vi "I2C Close.vi"(7 "I2C Channel (0)":u8, 8 "Error In":errorcluster, 11 "LINX Resource":T1) -> (0 "Error Out":errorcluster, 3 "LINX Resource":T1)   [LabVIEW 2014, in "LMH-LINX.lvlib"]
doc: "Close the specified I2C channel. Not all devices support or require this fuction. Most Wiring (Arduino) comaptible devices do not support this function. \n\nIf the current device does not support this function it will return a 'Function Not Supported' warning which should be handled by the users code."
uses:
  LMH-LINX.lvlib
  Private/Type Defs/LINX Ref.ctl
  Private/Type Defs/Platform.ctl
  Private/Type Defs/Interface.ctl
  Private/Device/Type Defs/LINX Device Config.ctl
  Private/Device/Type Defs/TCP Config.ctl
  Private/Device/Type Defs/Channels.ctl
  Private/Type Defs/Peripheral.ctl
  Private/Type Defs/Channel FGV States.ctl
  <vilib>/myRIO/Instrument Drivers/Onboard IO/I2C/typedefs/I2C Transfer Rate.ctl
  <vilib>/myRIO/Instrument Drivers/Onboard IO/I2C/I2C.lvlib
  <vilib>/myRIO/Instrument Drivers/Onboard IO/I2C/typedefs/I2C Configuration.ctl
  <vilib>/myRIO/Common/Instrument Driver Framework/myRIO v1.0/I2C/typedefs/I2C Channels Enum.ctl
  <vilib>/myRIO/Common/Instrument Driver Framework/Utilities/typedefs/Generic FPGA Reference.ctl
  <vilib>/myRIO/Common/Instrument Driver Framework/Utilities/typedefs/myRIO v1.0 Reference.ctl
  <vilib>/myRIO/Common/Instrument Driver Framework/Utilities/typedefs/Hardware Version Enum.ctl
  <vilib>/myRIO/Common/Instrument Driver Framework/Utilities/typedefs/myRIO Generic Hardware Reference.ctl
  <vilib>/myRIO/Instrument Drivers/Onboard IO/I2C/typedefs/I2C Reference.ctl
  Private/Device/Device.lvlib
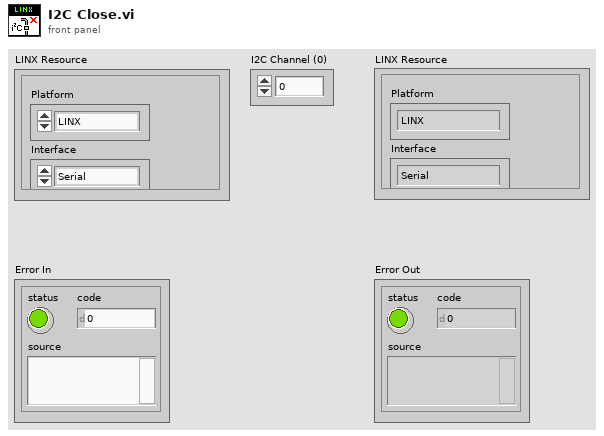
[diagram p1: front panel]
types:
  T1 = typedef "LMH-LINX.lvlib/LINX Ref.ctl" = cluster{"Platform":T2, "Interface":T3, "LINX Device Config":T4}
  T2 = typedef "LMH-LINX.lvlib/Platform.ctl" = enum16{"LINX", "myRIO"}
  T3 = typedef "LMH-LINX.lvlib/Interface.ctl" = enum16{"Serial", "TCP"}
  T4 = typedef "LMH-LINX.lvlib/Device.lvlib/LINX Device Config.ctl" = cluster{"Interface":T3, "COM Port":refnum<visa-resource-name>, "TCP Configuration":T5, "Device Family":u8, "Device ID":u8, "Device Name":string, "TCP Ref":refnum<k5>, "Channels":T6}
  T5 = typedef "LMH-LINX.lvlib/Device.lvlib/TCP Config.ctl" = cluster{"IP Address":string, "Port":u16}
  T6 = typedef "LMH-LINX.lvlib/Channels.ctl" = cluster{"DI":u8[], "DO":u8[], "AI":u8[], "AO":u8[], "PWM":u8[], "QE":u8[], "UART":u8[], "I2C 2":u8[], "SPI":u8[], "CAN":u8[], "Servo":u8[], "AI Ref (V)":dbl, "AO Ref (V)":dbl, "AO Resolution (Bits)":u8}
  T7 = typedef "LMH-LINX.lvlib/Peripheral.ctl" = enum8{"DI", "DO", "AI", "AO", "PWM", "QE", "UART", "I2C", "SPI", "CAN", "Servo"}
  T8 = typedef "LMH-LINX.lvlib/Channel FGV States.ctl" = enum16{"Initialize", "Get", "Set"}
  T9 = typedef "I2C.lvlib/I2C Reference.ctl" = cluster{"myRIO Reference":T10, "I2C Channels Enum":T14, "I2C Configuration":T15}
  T10 = typedef "myRIO Generic Hardware Reference.ctl" = cluster{"myRIO Model":T11, "myRIO Hardware Reference":T12}
  T11 = typedef "Hardware Version Enum.ctl" = enum16{"Unknown", "myRIO-1900", "myRIO-1950"}
  T12 = typedef "myRIO v1.0 Reference.ctl" = cluster{"Generic FPGA Reference":T13, "Allow multiple opens":bool}
  T13 = typedef "Generic FPGA Reference.ctl" = refnum<k20>
  T14 = typedef "I2C Channels Enum.ctl" = enum16{"Not Connected", "A/I2C", "B/I2C"}
  T15 = typedef "I2C.lvlib/I2C Configuration.ctl" = cluster{"I2C Transfer Rate":T16}
  T16 = typedef "I2C.lvlib/I2C Transfer Rate.ctl" = enum16{"Standard mode (100 kbps)", "Fast mode (400 kbps)"}
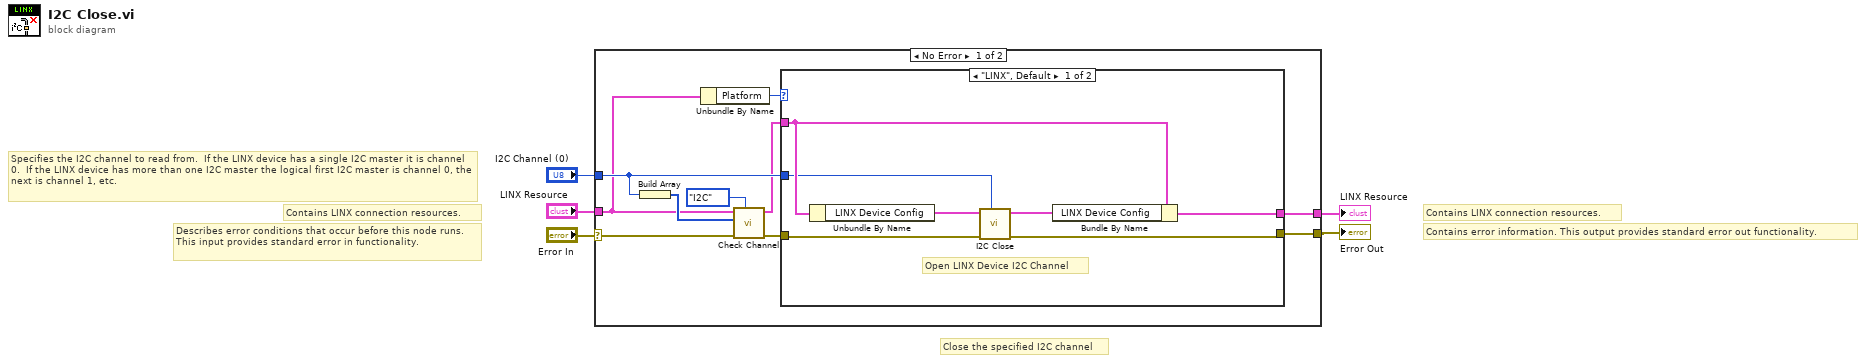
[diagram p0: block diagram]
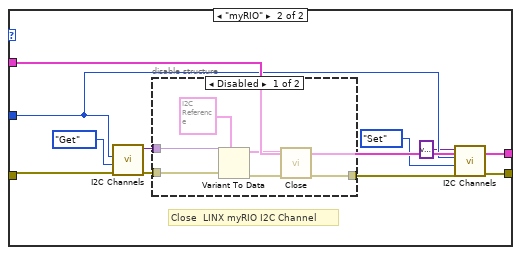
[diagram p2: hidden frame]
diagram:
  # "Specifies the I2C channel to read from.  If the LINX device has a single I2C master it is channel 0.  If the LINX device has more than one I2C master the logical first I2C master is channel 0, the next is channel 1, etc."
  # "Contains LINX connection resources."
  # "Contains error information. This output provides standard error out functionality."
  # "Contains LINX connection resources."
  # "Describes error conditions that occur before this node runs. This input provides standard error in functionality."
  # "Close the specified I2C channel"
  n1 = case shown="No Error" "Error In" {
    selector: "Error In" -> [w6 w40]
    tunnel: [w14 w40] -> w5
    tunnel: [w13 w39] -> w4
    tunnel: "I2C Channel (0)" -> [w9 _]
    tunnel: "LINX Resource" -> [w8 w39]
    frame No Error {
      n2 = Build Array(w9) -> (w12:u8[])
      n3 = Unbundle By Name(w8) -> ("Platform"=w15:T2)
      n4 = call "Check Channel.vi"("Peripheral"=Peripheral."I2C", "Error In"=w6, "Channels"=w12, "LINX Resource"=w8) -> ("Error Out"=w10:errorcluster, "LINX Resource"=w7:T1)  [unwired: 5 in, 1 out]
      n5 = case shown="\"LINX\", Default" w15 {
        tunnel: w10 -> [w17 w28]
        tunnel: w7 -> [w22 w32]
        tunnel: [w16 w31] -> w14
        tunnel: [w21 w32] -> w13
        tunnel: w9 -> [w18 w27]
        frame "LINX", Default {
          # "Open LINX Device I2C Channel"
          n6 = Unbundle By Name(w22) -> ("LINX Device Config"=w20:T4)
          n7 = call "I2C Close.vi"("I2C Channel"=w18, "Error In"=w17, "LINX Device Config"=w20) -> ("Error Out"=w16:errorcluster, "LINX Device Config"=w19:T4)  [unwired: 7 in]
          n8 = Bundle By Name(cluster=w22, "LINX Device Config"=w19) -> (w21:T1)
        }
        frame "myRIO" {
          # "Close  LINX myRIO I2C Channel"
          n9 = call "I2C Channels.vi"("Error In"=w28, "Channel State"=Channel_FGV_States."Get", "Channel Number"=w27) -> ("Error Out"=w25:errorcluster, "I2C Channel"=w26:variant)  [unwired: 7 in]
          n10 = disable-structure shown="Disabled" {
            disable-tunnel: w26 -> [w35 _]
            disable-tunnel: w25 -> [w34 _]
            disable-tunnel: [w33 _] -> w24
            frame Disabled {
              n11 = Variant To Data(error in=w34, type=T9 {"myRIO Reference"={"myRIO Model"=enum."Unknown", "myRIO Hardware Reference"={"Generic FPGA Reference"=refnum, "Allow multiple opens"=FALSE}}, "I2C Channels Enum"=enum."Not Connected", "I2C Configuration"={"I2C Transfer Rate"=enum."Standard mode (100 kbps)"}}, Variant=w35) -> (data=w37:T9, error out=w36:errorcluster)
              n12 = call <vilib>:"Close.vi"("error in (no error)"=w36, "I2C Ref In"=w37) -> ("error out"=w33:errorcluster)  [unwired: 9 in]
            }
            frame Enabled {
            }
          }
          n13 = call "I2C Channels.vi"("Error In"=w24, "Channel State"=Channel_FGV_States."Set", "Channel Number"=w27, "I2C Channel"=variant) -> ("Error Out"=w31:errorcluster)  [unwired: 6 in, 1 out]
        }
      }
    }
    frame Error {
    }
  }
  "Error Out" <- w5
  "LINX Resource" <- w4
